vi "10 LV - Who am I.vi"() -> ()   [LabVIEW 2020]
uses:
  client/User/User.lvclass
  client/Client/Client.lvclass
panel:
  out "Display Name":string
  out "User Email":string
  out "Org RID":string
  out "User RID":string
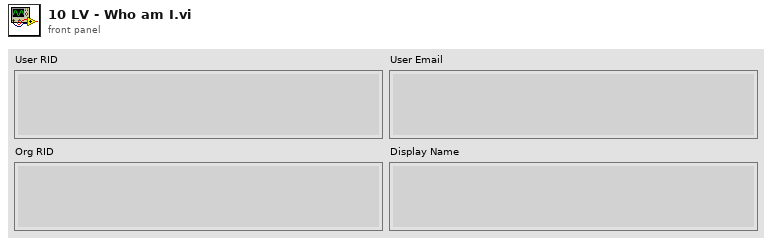
[diagram p1: front panel]
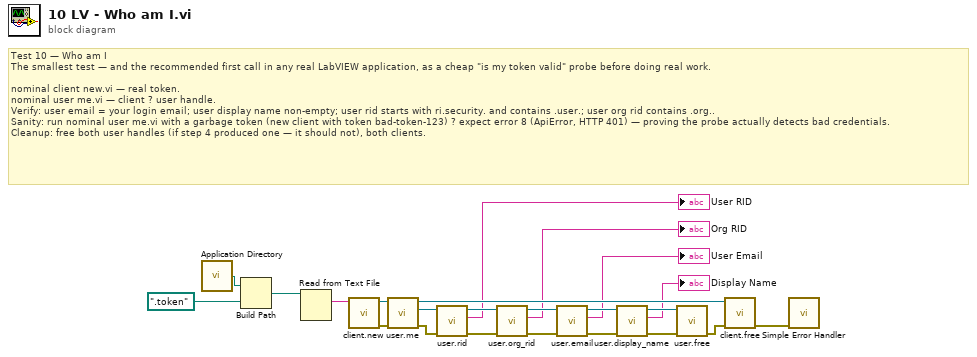
[diagram p0: block diagram]
diagram:
  # "Test 10 — Who am I\nThe smallest test — and the recommended first call in any real LabVIEW application, as a cheap \"is my token valid\" probe before doing real work.\n\nnominal client new.vi — real token.\nnominal user me.vi — client ? user handle.\nVerify: user email = your login email; user display name non-empty; user rid starts with ri.security. and contains .user.; user org rid contains .org..\nSanity: run nominal user me.vi with a garbage token (new client with token bad-token-123) ? expect error 8 (ApiError, HTTP 401) — proving the probe actually detects bad credentials.\nCleanup: free both user handles (if step 4 produced one — it should not), both clients."
  n1 = call <vilib>:"Application Directory.vi"() -> ("Application Directory"=w23:path)
  n2 = Build Path(base path=w23, name or relative path=path ".token") -> (appended path=w21:path)
  n3 = Read from Text File(file (use dialog)=w21) -> (text=w6:string)  [unwired: 3 in, 3 out]
  n4 = call "client.new.vi"("token"=w6) -> ("error out"=w8:errorcluster, "Client out"=w20:refnum<class "Client.lvclass">)  [unwired: 9 in]
  n5 = call "user.me.vi"("error in"=w8, "Client in"=w20) -> ("error out"=w7:errorcluster, "User"=w19:refnum<class "User.lvclass">, "Client out"=w9:refnum<class "Client.lvclass">)  [unwired: 7 in]
  n6 = call "user.rid.vi"("error in"=w7, "User in"=w19) -> ("error out"=w17:errorcluster, "user rid"=→"User RID":string, "User out"=w18:refnum<class "User.lvclass">)  [unwired: 7 in]
  n7 = call "user.org_rid.vi"("error in"=w17, "User in"=w18) -> ("error out"=w15:errorcluster, "user org id"=→"Org RID":string, "User out"=w16:refnum<class "User.lvclass">)  [unwired: 7 in]
  n8 = call "user.email.vi"("error in"=w15, "User in"=w16) -> ("error out"=w13:errorcluster, "user email"=→"User Email":string, "User out"=w14:refnum<class "User.lvclass">)  [unwired: 7 in]
  n9 = call "user.display_name.vi"("error in"=w13, "User in"=w14) -> ("error out"=w11:errorcluster, "display name"=→"Display Name":string, "User out"=w12:refnum<class "User.lvclass">)  [unwired: 7 in]
  n10 = call "user.free.vi"("error in"=w11, "User in"=w12) -> ("error out"=w10:errorcluster)  [unwired: 9 in]
  n11 = call "client.free.vi"("error in"=w10, "Client in"=w9) -> ("error out"=w1:errorcluster)  [unwired: 9 in]
  n12 = call <vilib>:"Simple Error Handler.vi"("error in (no error)"=w1) -> ()  [unwired: 4 in, 5 out]
